vi "Wait and Read from Oscilloscope.vi"(8 "error in (no error)":errorcluster, 9 "Waveform Width":u8(knob)=2 min=1 max=2 step=1 scale=0.0..2.0, 10 "data format":string, 11 "VISA resource name":refnum<visa-resource-name>) -> (0 "error out 2":errorcluster, 1 "dt (microseconds)":dbl, 2 "output waveform 2":waveform(dbl)(graph), 3 "VISA resource name 2":refnum<visa-resource-name>)   [LabVIEW 2018]
doc: "Use this template to build a VI to use as a subVI."
panel:
  out "substring":string
  out "read buffer":string
  out "length 2":i32
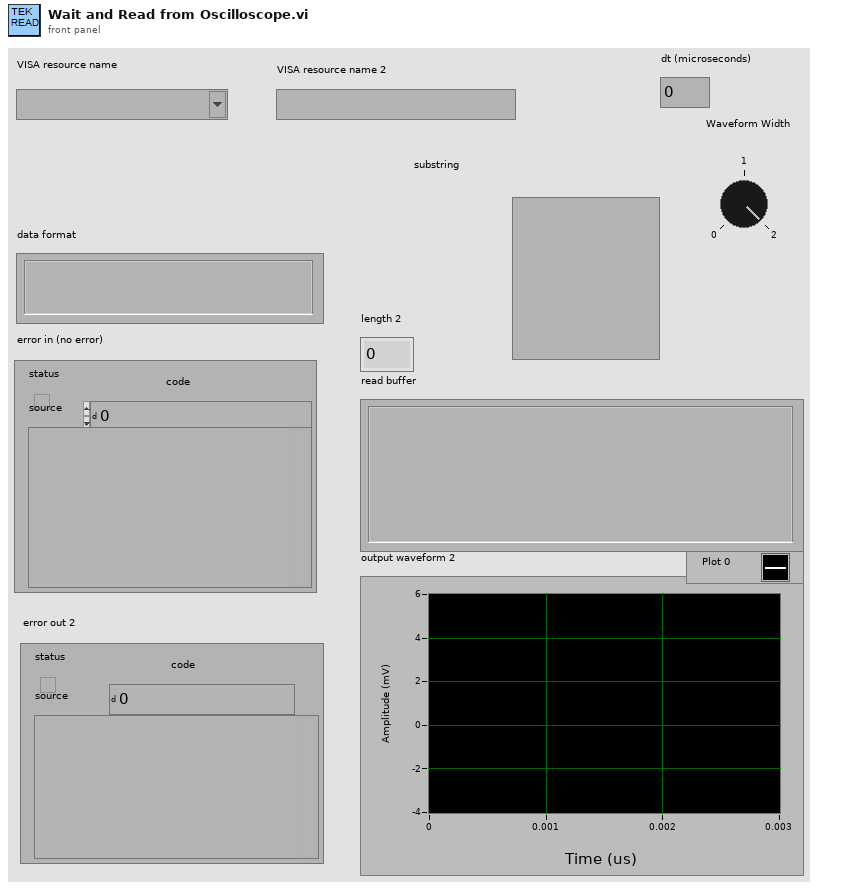
[diagram p1: front panel]
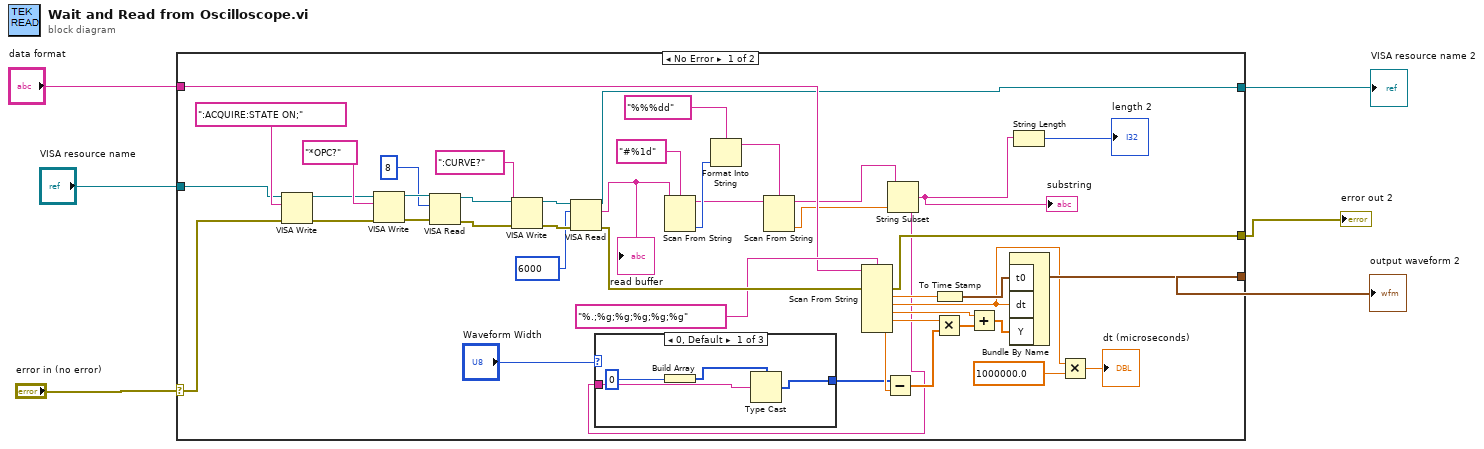
[diagram p0: block diagram]
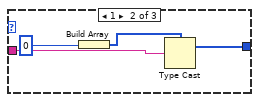
[diagram p2: hidden frame]
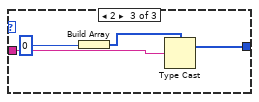
[diagram p3: hidden frame]
diagram:
  n1 = case shown="No Error" "error in (no error)" {
    selector: "error in (no error)" -> [w34 w64]
    tunnel: "VISA resource name" -> [w35 w63]
    tunnel: "data format" -> [w30 _]
    tunnel: [w25 w64] -> w2
    tunnel: [w26 _] -> w3
    tunnel: [w24 w63] -> w1
    frame No Error {
      n2 = VISA Write(VISA resource name=w35, write buffer=":ACQUIRE:STATE ON;", error in (no error)=w34) -> (VISA resource name out=w22:refnum<visa-resource-name>, error out=w21:errorcluster)  [unwired: 1 out]
      n3 = VISA Write(VISA resource name=w22, write buffer="*OPC?", error in (no error)=w21) -> (VISA resource name out=w20:refnum<visa-resource-name>, error out=w19:errorcluster)  [unwired: 1 out]
      n4 = VISA Read(VISA resource name=w20, byte count=u32 8, error in (no error)=w19) -> (VISA resource name out=w18:refnum<visa-resource-name>, error out=w17:errorcluster)  [unwired: 2 out]
      n5 = VISA Write(VISA resource name=w18, write buffer=":CURVE?", error in (no error)=w17) -> (VISA resource name out=w37:refnum<visa-resource-name>, error out=w38:errorcluster)  [unwired: 1 out]
      n6 = VISA Read(VISA resource name=w37, byte count=u32 6000, error in (no error)=w38) -> (VISA resource name out=w24:refnum<visa-resource-name>, read buffer=w43:string, error out=w44:errorcluster)  [unwired: 1 out]
      "read buffer" <- w43
      n7 = Scan From String(format string="#%1d", input string=w43) -> (remaining string=w15:string, output 1=w41:i32)  [unwired: 3 in, 2 out]
      n8 = Format Into String(format string="%%%dd", w41) -> (resulting string=w31:string)  [unwired: 2 in, 1 out]
      n9 = Scan From String(format string=w31, input string=w15) -> (remaining string=w14:string, output 1=w13:dbl)  [unwired: 3 in, 2 out]
      n10 = Scan From String(format string="%.;%g;%g;%g;%g;%g", input string=w30, error in=w44) -> (error out=w25:errorcluster, output 1=w32:dbl, output 2=w12:dbl, output 3=w27:dbl, output 4=w28:dbl, output 5=w29:dbl)  [unwired: 6 in, 2 out]
      n11 = String Subset(string=w14, length (rest)=w13) -> (substring=w8:string)  [unwired: 1 in]
      "substring" <- w8
      n12 = case shown="0, Default" "Waveform Width" {
        tunnel: w8 -> [w54 w58 w62]
        tunnel: [w53 w57 w61] -> w7
        frame 0, Default {
          n13 = Build Array(i8 0) -> (w51:i8[])
          n14 = Type Cast(type=w51, x=w54) -> (*(type *) &x=w53:i8[])
        }
        frame 1 {
          n15 = Build Array(i8 0) -> (w55:i8[])
          n16 = Type Cast(type=w55, x=w58) -> (*(type *) &x=w57:i8[])
        }
        frame 2 {
          n17 = Build Array(i16 0) -> (w59:i16[])
          n18 = Type Cast(type=w59, x=w62) -> (*(type *) &x=w61:i16[])
        }
      }
      n19 = Subtract(x=w7, y=w29) -> (x-y=w49:dbl[])
      n20 = Multiply(x=w28, y=w49) -> (x*y=w48:dbl[])
      n21 = To Time Stamp(1:w32) -> (0:w47:timestamp)
      n22 = Add(x=w27, y=w48) -> (x+y=w46:dbl[])
      n23 = Bundle By Name("t0"=w47, "dt"=w12, "Y"=w46) -> (w26:waveform(dbl))  [unwired: 1 in]
      n24 = String Length(string=w8) -> (length=→"length 2":i32)
      n25 = Multiply(x=w12, y=1000000.0) -> (x*y=→"dt (microseconds)":dbl)
    }
    frame Error {
    }
  }
  "error out 2" <- w2
  "output waveform 2" <- w3
  "VISA resource name 2" <- w1
